vi "GMLAN TesterPresent.vi"(8 "error in (no error)":errorcluster, 10 "Parameter":T1, 11 "diag ref in":T2) -> (0 "error out":errorcluster, 1 "success?":bool, 3 "diag ref out":T2)   [LabVIEW 2013, in "GMLAN.lvlib"]
uses:
  GMLAN.lvlib
  <vilib>/Automotive Diagnostic Command Set/Diagnostic Transport.llb/Diag Reference.ctl
  <vilib>/Automotive Diagnostic Command Set/Diagnostic Transport.llb/Transport Protocol Selector.ctl
  <vilib>/Automotive Diagnostic Command Set/Diagnostic Transport.llb/Diag CAN Frame Log.ctl
  _SubVIs/TesterPresent_Parameter.ctl
  <vilib>/Automotive Diagnostic Command Set/Diagnostic Transport.llb/Apply Diagnostic Error.vi
  <vilib>/Automotive Diagnostic Command Set/Diagnostic Transport.llb/Diag Globals.vi
  <vilib>/Automotive Diagnostic Command Set/Diagnostic Transport.llb/Diagnostic Service Send.vi
  <vilib>/addons/Automotive Diagnostic Command Set/NI_Automotive Diagnostic Command Set.lvlib
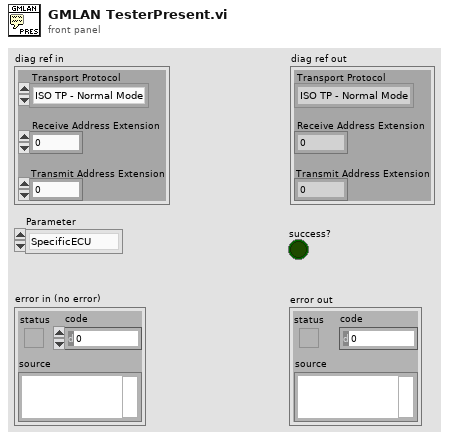
[diagram p1: front panel]
types:
  T1 = typedef "GMLAN.lvlib/TesterPresent_Parameter.ctl" = enum8{"SpecificECU", "EntireNetwork"}
  T2 = typedef "NI_Automotive Diagnostic Command Set.lvlib/Diag Reference.ctl" = cluster{"Diag CAN Handle":u32, "Transport Protocol":T3, "Receive Address Extension":u8, "Transmit Address Extension":u8, "Receive CAN Id":u32, "Transmit CAN Id":u32, "Diag CAN Queue":refnum<queue>, "Log Frames ?":bool, "My TP Address":u8, "Other TP Address":u8, "T1":u16, "T2":u16, "T3":u16, "T4":u16, "Tx SN":u8, "Block Size":u8, "Rx SN":u8, "VW TP Initialized?":bool, "Tx block no":u8, "baud rate":u32, "Interface":string, "Channel Diag CAN Handle":u32, "UDP Connection ID":refnum<k16>, "TCP Connection ID":refnum<k5>, "Target IP Addr":u32, "Source Address":u16, "Target Address":u16, "Send Header NACK?":bool, "DLL Handle":u32, "NAD":u8, "Time Stamp read first":dbl, "Time Stamp read last":dbl, "Time Stamp write first":dbl, "Time Stamp write last":dbl, "Time Stamp write":dbl, "Time Stamp read":dbl}
  T3 = typedef "NI_Automotive Diagnostic Command Set.lvlib/Transport Protocol Selector.ctl" = enum16{"ISO TP - Normal Mode", "ISO TP - Mixed Mode", "VW TP 2.0", "Diagnostics on IP", "ISO TP LIN"}
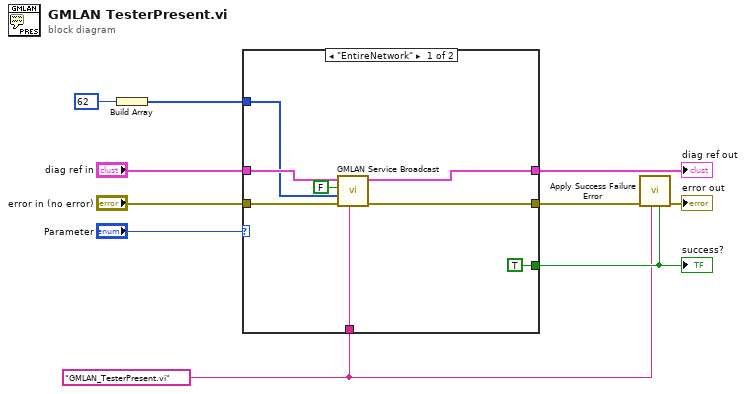
[diagram p0: block diagram]
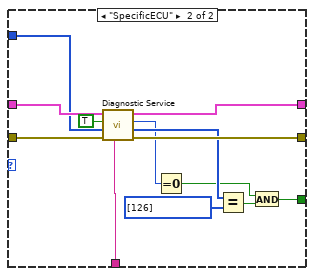
[diagram p2: hidden frame]
diagram:
  w2 = "GMLAN_TesterPresent.vi" ("error source")
  n1 = Build Array(u8 62) -> (w5:u8[])
  n2 = case shown="\"EntireNetwork\"" "Parameter" {
    tunnel: "error in (no error)" -> [w18 w31]
    tunnel: [w16 w30] -> w9
    tunnel: [w15 w28] -> w8
    tunnel: "diag ref in" -> [w17 w27]
    tunnel: w5 -> [w14 w26]
    tunnel: [TRUE w24] -> w3
    tunnel: w2 -> [w11 w23]
    frame "EntireNetwork" {
      n3 = call "GMLAN Service Broadcast.vi"("error source"=w11, "error in (no error)"=w18, "data in"=w14, "require response?"=FALSE, "diag ref in"=w17) -> ("error out"=w16:errorcluster, "diag ref out"=w15:T2)  [unwired: 3 in, 2 out]
    }
    frame "SpecificECU" {
      n4 = call <vilib>:"Diagnostic Service.vi"("error source"=w23, "error in (no error)"=w31, "data in"=w26, "require response?"=TRUE, "diag ref in"=w27) -> ("error out"=w30:errorcluster, "data out"=w29:u8[], "error code"=w25:u8, "diag ref out"=w28:T2)  [unwired: 1 in, 2 out]
      n5 = Equal To 0?(x=w25) -> (x = 0?=w20:bool)
      n6 = Equal?(x=w29, y=u8[] [126]) -> (x = y?=w21:bool)
      n7 = And(x=w20, y=w21) -> (x .and. y?=w24:bool)
    }
  }
  "success?" <- w3
  "diag ref out" <- w8
  n8 = call <vilib>:"Apply Success Failure Error.vi"("success code"=w3, "error source"=w2, "error in (no error)"=w9) -> ("error out"=→"error out":errorcluster)  [unwired: 8 out]
